vi "ELVIS III v1.0 RPC Unregister Abort.vi"(8 "error in (no error)":errorcluster, 11 "Session":u32) -> (0 "error out":errorcluster)   [LabVIEW 2021]
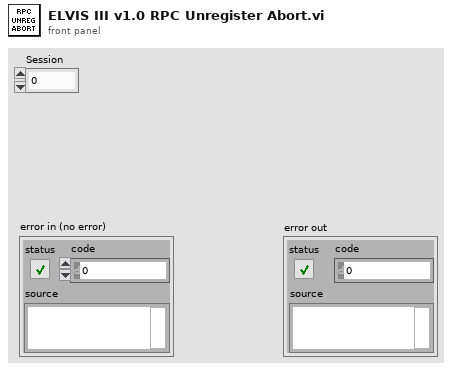
[diagram p1: front panel]
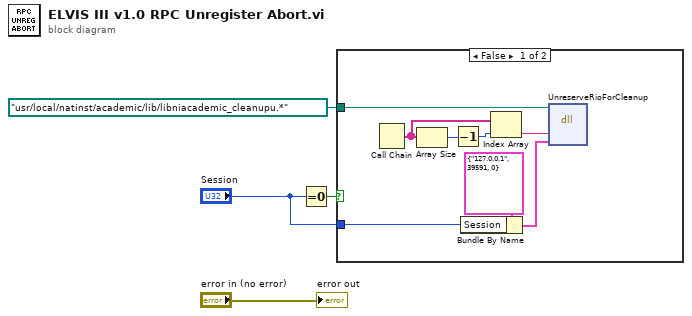
[diagram p0: block diagram]
diagram:
  n1 = Equal To 0?(x="Session") -> (x = 0?=w1:bool)
  n2 = case shown="False" w1 {
    tunnel: "Session" -> [w6 _]
    tunnel: path "/usr/local/natinst/academic/lib/libniacademic_cleanupu.*" ("path in") -> [w12 _]
    frame False {
      n3 = Call Chain() -> (call chain=w9:string[])
      n4 = Array Size(array=w9) -> (size(s)=w11:i32)
      n5 = Decrement(x=w11) -> (x-1=w10:i32)
      n6 = Bundle By Name(cluster=cluster{"IP":string, "Port":i32, "Session":u32} {"IP"="127.0.0.1", "Port"=39591, "Session"=0}, "Session"=w6) -> (w5:cluster{"IP":string, "Port":i32, "Session":u32})
      n7 = Index Array(array=w9, index=w10) -> (element=w8:string)
      n8 = dll-call lib="?" fn="UnreserveRioForCleanup"(path in=w12, "topVIName"=w8, "resourcesInfo"=w5) -> ()  [unwired: 5 in, 2 out]
    }
    frame True {
      # "Session is invalid i.e. call from rpc server"
    }
  }
  "error out" <- "error in (no error)"
